vi "ApplicationConfiguration (FGV).vi"(7 "FGV Action":T1, 8 "Error in":errorcluster, 11 "App Configuration in":T2) -> (0 "Error out":errorcluster, 3 "App Configuration out":T2)   [LabVIEW 2019]
uses:
  #cluster_AppConfiguration.ctl
  #enum_FGVAction.ctl
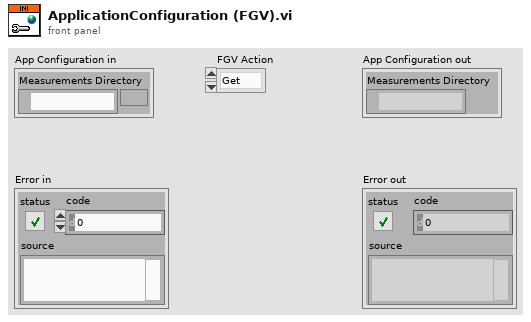
[diagram p1: front panel]
types:
  T1 = typedef "#enum_FGVAction.ctl" = enum16{"Get", "Set"}
  T2 = typedef "#cluster_AppConfiguration.ctl" = cluster{"Measurements Directory":path}
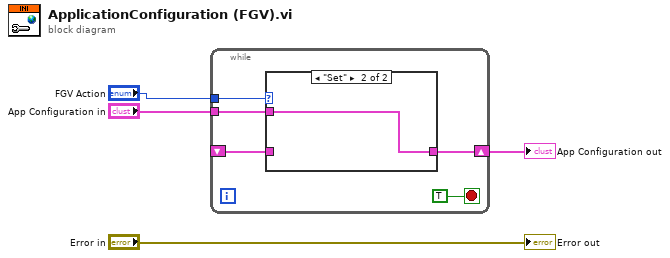
[diagram p0: block diagram]
diagram:
  n1 = while {
    shift-right: [w6] -> w4
    shift-left: _ -> [w7]
    tunnel: "FGV Action" -> [w8]
    tunnel: "App Configuration in" -> [w5]
    stop <- TRUE stop-if-true
    n2 = case shown="\"Set\"" w8 {
      tunnel: w7 -> [w10 _]
      tunnel: [w10 w11] -> w6
      tunnel: w5 -> [_ w11]
      frame "Get", Default {
      }
      frame "Set" {
      }
    }
  }
  "App Configuration out" <- w4
  "Error out" <- "Error in"
